vi "DMD_stop.vi"(11 "reference out":refnum<k24>) -> (0 "error out":errorcluster)   [LabVIEW 2017]
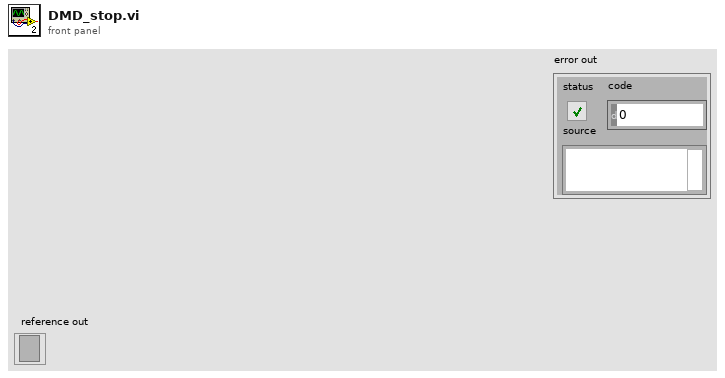
[diagram p1: front panel]
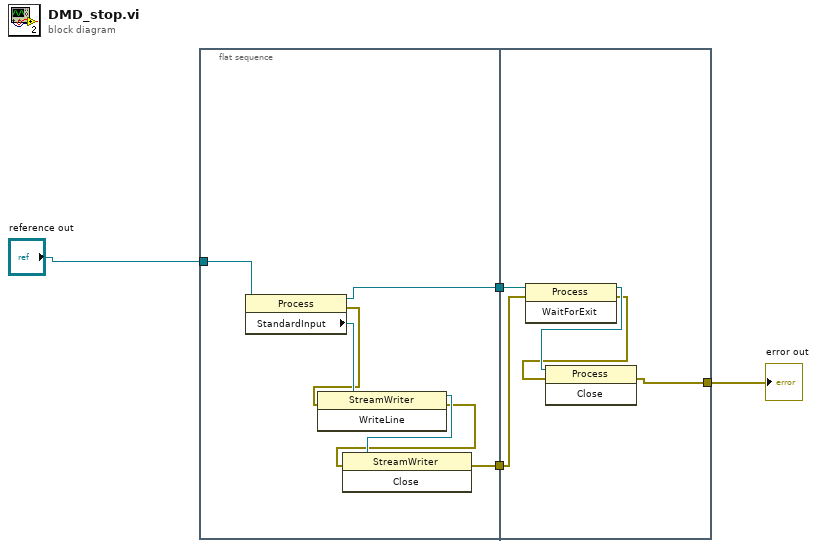
[diagram p0: block diagram]
diagram:
  n1 = flat-sequence {
    tunnel: [w9] -> w4
    tunnel: "reference out" -> [w8]
    tunnel: [w5] -> w2
    tunnel: w4 -> [w16]
    tunnel: w2 -> [w14]
    tunnel: [w12] -> w1
    frame #0 {
      n2 = property class="Process"(reference=w8) -> (reference out=w9:refnum<k24>, error out=w7:errorcluster, "StandardInput"=w11:refnum<k24>)  [unwired: 1 in]
      n3 = invoke class="StreamWriter" method="WriteLine"(reference=w11, error in=w7) -> (reference out=w10:refnum<k24>, error out=w6:errorcluster)  [unwired: 1 in, 1 out]
      n4 = invoke class="StreamWriter" method="Close"(reference=w10, error in=w6) -> (error out=w5:errorcluster)  [unwired: 1 in, 2 out]
    }
    frame #1 {
      n5 = invoke class="Process" method="WaitForExit"(reference=w16, error in=w14) -> (reference out=w15:refnum<k24>, error out=w13:errorcluster)  [unwired: 1 in, 1 out]
      n6 = invoke class="Process" method="Close"(reference=w15, error in=w13) -> (error out=w12:errorcluster)  [unwired: 1 in, 2 out]
    }
  }
  "error out" <- w1
